vi "Launch Actors from Core.vi"(8 "error in (no error)":errorcluster, 11 "Core in":refnum<class "Core.lvclass">) -> (0 "error out":errorcluster, 3 "Core out":refnum<class "Core.lvclass">)   [LabVIEW 2019, in "Core.lvlib" / "Core.lvclass"]
uses:
  Core.lvclass
  C:/Projekty/_Wewnetrzne/PC_ActorFramework/07_Program/LABVIEW/02_Source/Modules/ModuleAbstract/ModuleAbstract.lvclass
  SubModules/ErrorLog/ErrorLog.lvclass
  SubModules/EventLog/EventLog.lvclass
  ModuleAbstract/ModuleAbstract.lvclass
  C:/Projekty/_Wewnetrzne/PC_ActorFramework/07_Program/LABVIEW/02_Source/SubModules/LogsAbstract/LogsAbstract.lvclass
  C:/Program Files (x86)/National Instruments/LabVIEW 2019/vi.lib/MGI/Monitored Actor/Monitored Actor/Monitored Actor/Monitored Actor.lvclass
  C:/Program Files (x86)/National Instruments/LabVIEW 2019/vi.lib/ActorFramework/Actor/Actor.lvclass
  SubModules/LogsAbstract/LogsAbstract.lvclass
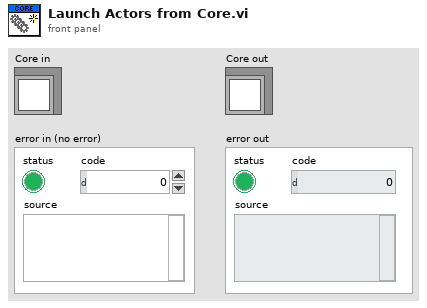
[diagram p1: front panel]
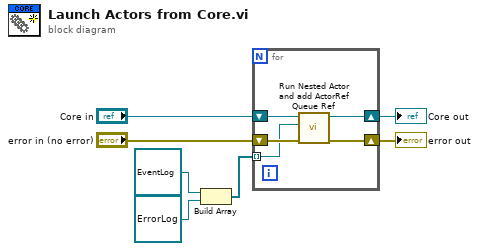
[diagram p0: block diagram]
diagram:
  n1 = Build Array(refnum<class "EventLog.lvclass"> refnum ("EventLog.lvlib:EventLog.lvclass"), refnum<class "ErrorLog.lvclass"> refnum ("ErrorLog.lvlib:ErrorLog.lvclass")) -> (w2:refnum<class "LogsAbstract.lvclass">[])
  n2 = for {
    tunnel: w2 -> [w9] mode=indexing
    shift-right: [w11] -> w6
    shift-left: "error in (no error)" -> [w12]
    shift-right: [w10] -> w5
    shift-left: "Core in" -> [w8]
    n3 = call "Run Nested Actor and add ActorRef Queue Ref.vi"("error in (no error)"=w12, "Nested Module"=w9, "LaunchingModule In"=w8) -> ("error out"=w11:errorcluster, "LaunchingModule In"=w10:refnum<class "Core.lvclass">)  [unwired: 6 in, 1 out]
  }
  "error out" <- w6
  "Core out" <- w5
